vi "二维数组查找元素_整数.vi"(8 "error in (no error)":errorcluster caption="错误输入（无错误）", 10 "元素":i32[](array[numeric]), 11 "二维数组":i32[][](array[numeric])) -> (0 "error out":errorcluster caption="错误输出", 1 "存在？":bool, 3 "位置":i32[](array[numeric]))   [LabVIEW 2014]
doc: "该模板用于创建子VI。"
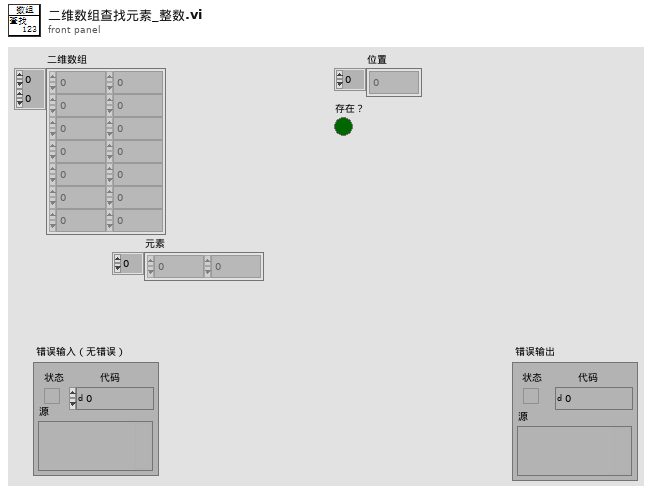
[diagram p1: front panel]
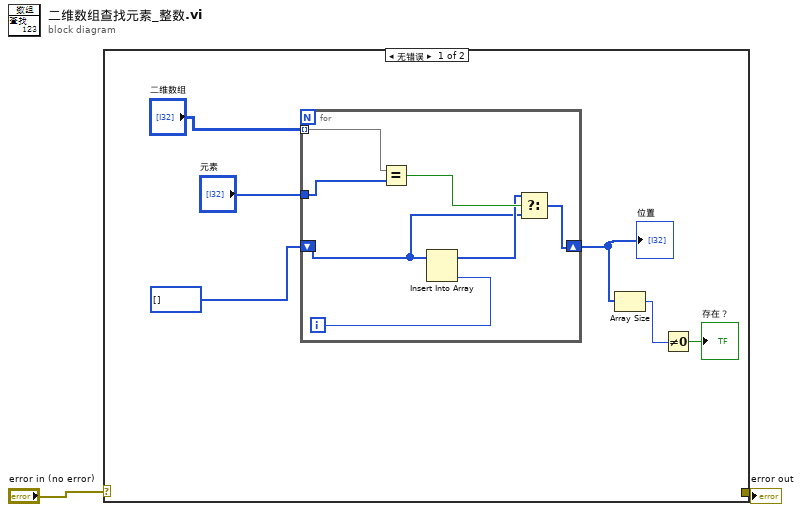
[diagram p0: block diagram]
diagram:
  n1 = case shown="无错误" "error in (no error)" {
    selector: "error in (no error)" -> [_ w16]
    tunnel: [_ w16] -> w1
    frame No Error {
      n2 = for {
        tunnel: "二维数组" -> [w15] mode=indexing
        tunnel: "元素" -> [w14]
        shift-right: [w9] -> w5
        shift-left: i32[] [] ("数组") -> [w10]
        i -> [w13]
        n3 = Equal?(x=w15, y=w14) -> (x = y?=w12:bool)
        n4 = Insert Into Array(array=w10, new element=w13) -> (w11:i32[])  [unwired: 1 in]
        n5 = Select(t=w11, s=w12, f=w10) -> (s? t:f=w9:i32[])
      }
      "位置" <- w5
      n6 = Array Size(array=w5) -> (size(s)=w4:i32)
      n7 = Not Equal To 0?(x=w4) -> (x != 0?=→"存在？":bool)
    }
    frame Error {
    }
  }
  "error out" <- w1
